vi "p2.vi"() -> ()   [LabVIEW 2023, in "d1.lvlib"]
uses:
  d1.lvlib
  <vilib>/regexp/Match Regular Expression.xnode
  AOC/AOC.lvlib
panel:
  in  "Input":string="sixrrmlkptmc18zhvninek\njcb82eightwond\ntwofourthree778nineeight\nsqpxs1cgcrmctlgqvzxbcjzgr\nnqkjxbmbpkz9eight8\none6fourfiveqndtrvgkkgthppnine\nzbrbdpbfcfxcqq5oneninejfgqpkfn\nhvlstzgvmjfivefourqjqtxdjmbxfour4four2\n13dzbmbtl6\nfourone2pmlxzzbmnfxg2\n3fourrbvvlrsrbb2858\nvlz4six89\n75threeb\nfourp783fiveseventhree\n2gxvcbsmn6\n896\ndnblxtxxpstlsix56\n4fivecl185\nonefk8sdljtfv37zsxsxrv7qvrpnmd\nfourdvhzp7foursix\nseventwonineseven27jbrqpxfx8\n1threenine241gnrdfqn5\nsixnrsqdgmkvs7sevenkgjgtglmdq9dkdzsdqmq2nptbxnxghm\nllbkdcpxkg1tnmnmrbskpdb\nzb7nvjz1eighttwo6nine\n5threeeightwor\ntgjmdbr4sixone5\n4twoseven7tjmklbl\nlt2vqg..."
  in  "Example":string="two1nine\neightwothree\nabcone2threexyz\nxtwone3four\n4nineeightseven2\nzoneight234\n7pqrstsixteen"
  in  "Example?":bool
  out "Answer":i64=55291
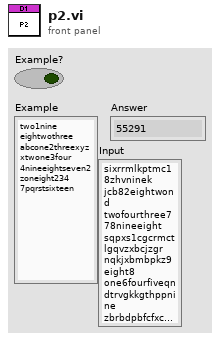
[diagram p1: front panel]
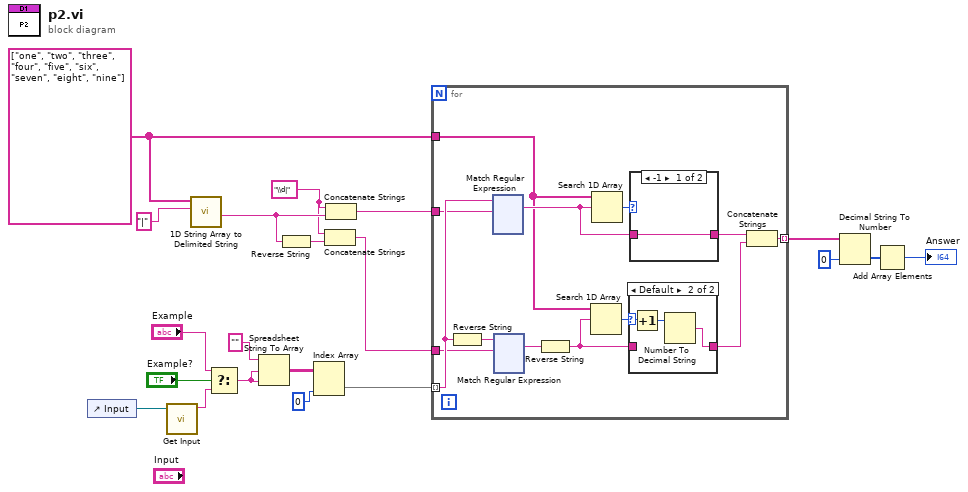
[diagram p0: block diagram]
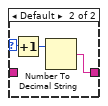
[diagram p2: hidden frame]
diagram:
  w5 = "\\d|" ("delimiter (Tab)")
  w3 = string[] ["one", "two", "three", "four", "five", "six", "seven", "eight", "nine"] ("regular expression")
  n1 = control-ref of="Input"() -> (w1:refnum<vi>)
  n2 = call "Get Input.vi"("Input ref"=w1) -> ("Input"=w19:string)  [unwired: 10 in]
  n3 = call <vilib>:"1D String Array to Delimited String.vi"("delimiter"="|" ("delimiter (Tab)"), "string array"=w3) -> ("delimited string"=w7:string)  [unwired: 9 in]
  n4 = Select(t="Example", s="Example?", f=w19) -> (s? t:f=w17:string)
  n5 = Spreadsheet String To Array(format string="", spreadsheet string=w17, array type (2D Dbl)=w17) -> (array=w11:string[][])  [unwired: 1 in]
  n6 = Reverse String(1:w7) -> (0:w6:string)
  n7 = Index Array(array=w11, index (col)=0 ("disabled index (col)")) -> (element=w9:string[])  [unwired: 1 in]
  n8 = Concatenate Strings(w5, w6) -> (w4:string)
  n9 = Concatenate Strings(w5, w7) -> (w8:string)
  n10 = for {
    tunnel: w9 -> [w33] mode=indexing
    tunnel: [w31] -> w16 mode=indexing
    tunnel: w8 -> [w30]
    tunnel: w4 -> [w29]
    tunnel: w3 -> [w21]
    n11 = Reverse String(1:w33) -> (0:w32:string)
    n12 = xnode "Match Regular Expression"("input string"=w33, "regular expression"=w30) -> ("whole match"=w23:string)  [unwired: 4 in, 4 out]
    n13 = xnode "Match Regular Expression"("input string"=w32, "regular expression"=w29) -> ("whole match"=w28:string)  [unwired: 4 in, 4 out]
    n14 = Reverse String(1:w28) -> (0:w26:string)
    n15 = Search 1D Array(1D array=w21, element=w26) -> (index of element=w27:i32)  [unwired: 1 in]
    n16 = Search 1D Array(1D array=w21, element=w23) -> (index of element=w24:i32)  [unwired: 1 in]
    n17 = case shown="Default" w27 {
      selector: w27 -> [_ w41]
      tunnel: w26 -> [w38 _]
      tunnel: [w38 w39] -> w25
      frame -1 {
      }
      frame Default {
        n18 = Increment(x=w41) -> (x+1=w40:i32)
        n19 = Number To Decimal String(number=w40) -> (decimal integer string=w39:string)  [unwired: 1 in]
      }
    }
    n20 = case shown="-1" w24 {
      selector: w24 -> [_ w37]
      tunnel: w23 -> [w34 _]
      tunnel: [w34 w35] -> w22
      frame -1 {
      }
      frame Default {
        n21 = Increment(x=w37) -> (x+1=w36:i32)
        n22 = Number To Decimal String(number=w36) -> (decimal integer string=w35:string)  [unwired: 1 in]
      }
    }
    n23 = Concatenate Strings(w22, w25) -> (w31:string)
  }
  n24 = Decimal String To Number(string=w16, default (0L)=i64 0 ("default (0 I32)")) -> (number=w14:i64[])  [unwired: 1 in, 1 out]
  n25 = Add Array Elements(numeric array=w14) -> (sum=→"Answer":i64)
